vi "getCursorPropertiesFromUser.vi"(8 "error in (no error)":errorcluster, 11 "Cursor Properties in":T1={"font"={"Font Name"="Arial", "Size"=16, "Strikeout?"=FALSE, "Italic?"=FALSE, "Underline?"=FALSE, "Outline?"=FALSE, "Shadow"=FALSE, "Bold?"=FALSE}, "size"=2, "time format (%H:%M:%S)"="%H:%M:%S", "Vertical Line?"=TRUE, "Horizontal Line?"=TRUE, "alignment(left, top)"={"Horizontal"=enum."center", "Vertical"=enum."center"}, "TextFormat"="%3$s\\n%2$.2f", "Timestamp"=enum."at BOTTOM"} {"size" min=1 max=50}) -> (0 "error out":errorcluster, 2 "ok":bool, 3 "Cursor Properties out":T1={"font"={"Font Name"="Arial", "Size"=16, "Strikeout?"=FALSE, "Italic?"=FALSE, "Underline?"=FALSE, "Outline?"=FALSE, "Shadow"=FALSE, "Bold?"=FALSE}, "size"=2, "time format (%H:%M:%S)"="%H:%M:%S", "Vertical Line?"=TRUE, "Horizontal Line?"=TRUE, "alignment(left, top)"={"Horizontal"=enum."center", "Vertical"=enum."center"}, "TextFormat"="%3$s\\n%2$.2f", "Timestamp"=enum."at BOTTOM"} {"size" min=1 max=50})   [LabVIEW 2017, in "QControl_Graph.lvclass"]
uses:
  QControl_Graph.lvclass
  Cursor Properties.ctl
  Font.ctl
  Alignment.ctl
  Alignment.Horizontal.ctl
  Alignment.Vertical.ctl
  selectCursorProperties.vi
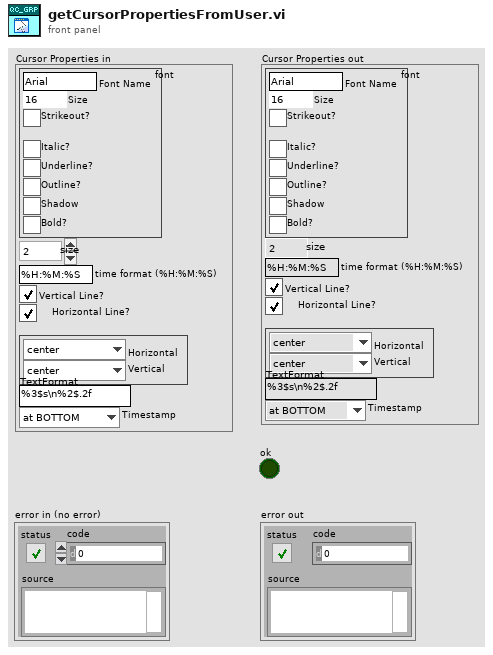
[diagram p1: front panel]
types:
  T1 = typedef "QControl_Graph.lvclass/Cursor Properties.ctl" = cluster{"font":T2, "size":i16, "time format (%H:%M:%S)":string, "Vertical Line?":bool, "Horizontal Line?":bool, "alignment(left, top)":T3, "TextFormat":string, "Timestamp":enum16{"at TOP", "at BOTTOM", "none"}}
  T2 = typedef "QControl_Graph.lvclass/Font.ctl" = cluster{"Font Name":string, "Size":i16, "Strikeout?":bool, "Italic?":bool, "Underline?":bool, "Outline?":bool, "Shadow":bool, "Bold?":bool}
  T3 = typedef "QControl_Graph.lvclass/Alignment.ctl" = cluster{"Horizontal":T4, "Vertical":T5}
  T4 = typedef "QControl_Graph.lvclass/Alignment.Horizontal.ctl" = enum16{"left", "center", "right"}
  T5 = typedef "QControl_Graph.lvclass/Alignment.Vertical.ctl" = enum16{"top", "center", "bottom"}
  T6 = enum32{"Invalid", "Standard", "Closed", "Hidden", "Minimized", "Maximized"}
  T7 = enum32{"Invalid", "Default", "Floating", "Floating/Auto-Hide", "Modal"}
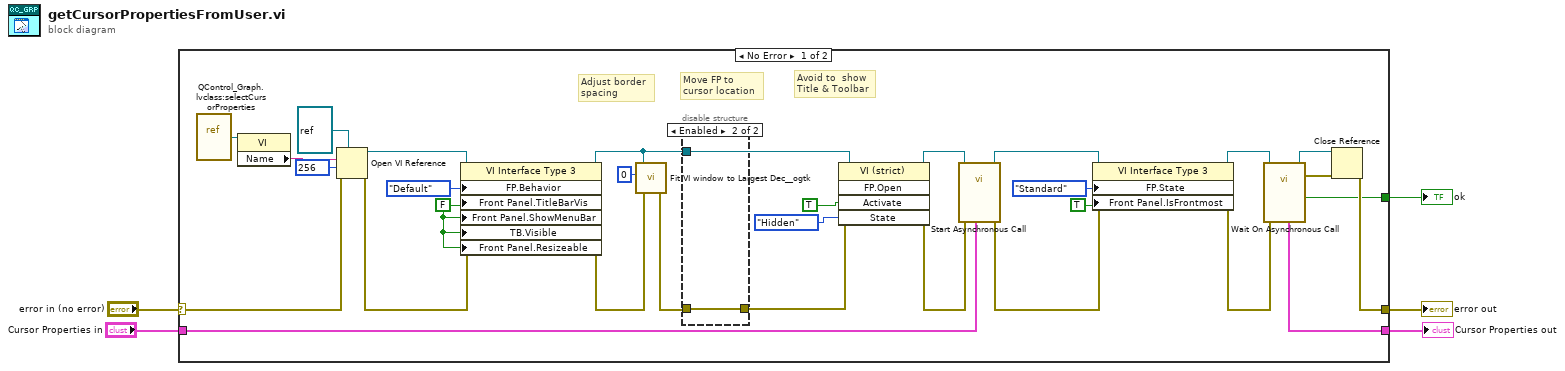
[diagram p0: block diagram]
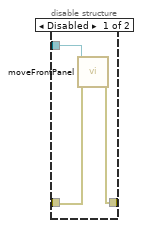
[diagram p2: hidden frame]
diagram:
  n1 = case shown="No Error" "error in (no error)" {
    selector: "error in (no error)" -> [w14 w41]
    tunnel: [w13 w41] -> w4
    tunnel: [w12 w40] -> w2
    tunnel: [w11 _] -> w3
    tunnel: "Cursor Properties in" -> [w6 w40]
    frame No Error {
      w34 = FALSE ("Front Panel Window:Title Bar Visible")
      # "Adjust border\nspacing"
      # "Move FP to \ncursor location"
      # "Avoid to  show\nTitle & Toolbar"
      n2 = vi-ref "QControl_Graph.lvclass:selectCursorProperties.vi"() -> (w28:refnum<vi>)
      n3 = property class="VI"(reference=w28) -> ("Name"=w27:string)  [unwired: 1 in, 2 out]
      n4 = Open VI Reference(type specifier VI Refnum (for type only)=refnum<vi> refnum, vi path=w27, options=256, error in (no error)=w14) -> (vi reference=w24:refnum<vi>, error out=w23:errorcluster)  [unwired: 2 in]
      n5 = property class="VI Interface Type 3"(reference=w24, error in=w23, "FP.Behavior"=T7."Default" ("Front Panel Window:Behavior"), "Front Panel.TitleBarVis"=w34, "Front Panel.ShowMenuBar"=w34, "TB.Visible"=w34, "Front Panel.Resizeable"=w34) -> (reference out=w7:refnum<vi>, error out=w9:errorcluster)
      n6 = call <userlib>:"Fit VI window to Largest Dec__ogtk.vi"("error in (no error)"=w9, "border spacing (2 px)"=0, "VI Ref (calling VI)"=w7) -> ("error out"=w8:errorcluster)  [unwired: 3 in, 1 out]
      n7 = disable-structure shown="Enabled" {
        disable-tunnel: [w38 w39] -> w30
        disable-tunnel: w8 -> [w37 w39]
        disable-tunnel: w7 -> [w36 _]
        frame Disabled {
          n8 = call "moveFrontPanel.vi"("error in (no error)"=w37, "VI in"=w36) -> ("error out"=w38:errorcluster)  [unwired: 8 in, 1 out]
        }
        frame Enabled {
        }
      }
      n9 = invoke class="VI (strict)" method="FP.Open"(reference=w7, error in=w30, "Activate"=TRUE ("Activate?"), "State"=T6."Hidden") -> (reference out=w22:refnum<vi>, error out=w20:errorcluster)  [unwired: 1 in, 3 out]
      n10 = call-by-ref "Start Asynchronous Call"(reference=w22, error in=w20, "Cursor Properties in"=w6) -> (reference out=w21:refnum<vi>, error out=w19:errorcluster)  [unwired: 9 in, 2 out]
      n11 = property class="VI Interface Type 3"(reference=w21, error in=w19, "FP.State"=T6."Standard" ("Front Panel Window:State"), "Front Panel.IsFrontmost"=TRUE ("Activate?")) -> (reference out=w18:refnum<vi>, error out=w17:errorcluster)
      n12 = call-by-ref "Wait On Asynchronous Call"(reference=w18, error in=w17) -> (reference out=w16:refnum<vi>, error out=w15:errorcluster, "ok"=w11:bool, "Cursor Properties out"=w12:T1)  [unwired: 10 in]
      n13 = Close Reference(reference=w16, error in (no error)=w15) -> (error out=w13:errorcluster)
    }
    frame Error {
    }
  }
  "error out" <- w4
  "ok" <- w3
  "Cursor Properties out" <- w2
